vi "APS-7050 Wrapper.vi"(7 "States":T3=enum."Config", 8 "error in":errorcluster, 9 "Enable Output":bool=TRUE, 10 "Setting":T2, 11 "Alias":string="ACPS") -> (0 "error out":errorcluster, 1 "Connect?":bool, 2 "output cluster":T1, 3 "Measurement":dbl=nan)   [LabVIEW 2021, in "MIO Wrappers.lvlib"]
doc: "This is a wrapper to support Keysight N6700C."
uses:
  MIO Wrappers.lvlib
  Controls/PS States.ctl
  Load INI/Controls/Instruments_Data.ctl
  <instrlib>/APS-7000 Series/APS-7000 Series.lvlib
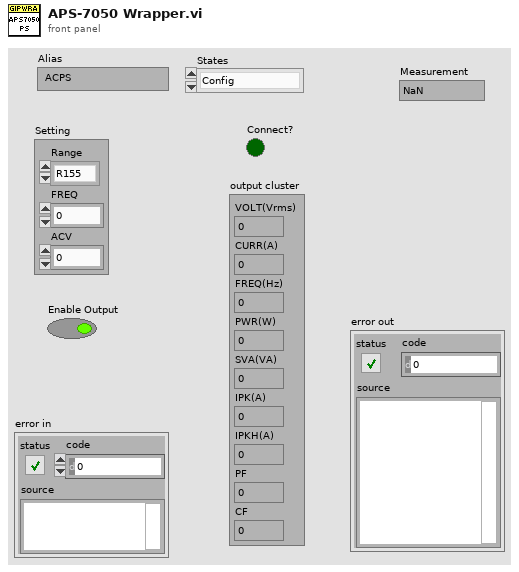
[diagram p1: front panel]
types:
  T1 = cluster{"VOLT(Vrms)":dbl, "CURR(A)":dbl, "FREQ(Hz)":dbl, "PWR(W)":dbl, "SVA(VA)":dbl, "IPK(A)":dbl, "IPKH(A)":dbl, "PF":dbl, "CF":dbl}
  T2 = cluster{"Range":enum16{"R155", "R310", "R600", "AUTO"}, "FREQ":dbl, "ACV":dbl}
  T3 = typedef "MIO Wrappers.lvlib/PS States.ctl" = enum16{"Init", "Config", "Enable Output", "Measure", "Close"}
  T4 = typedef "Instruments_Data.ctl" = cluster{"Alias":string, "Resource ":string}
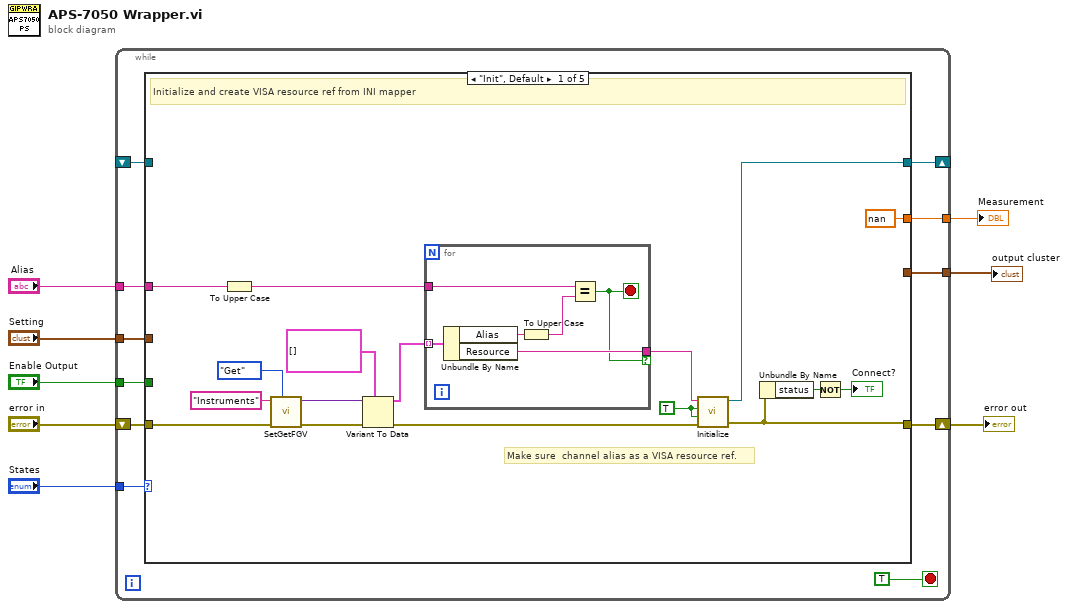
[diagram p0: block diagram]
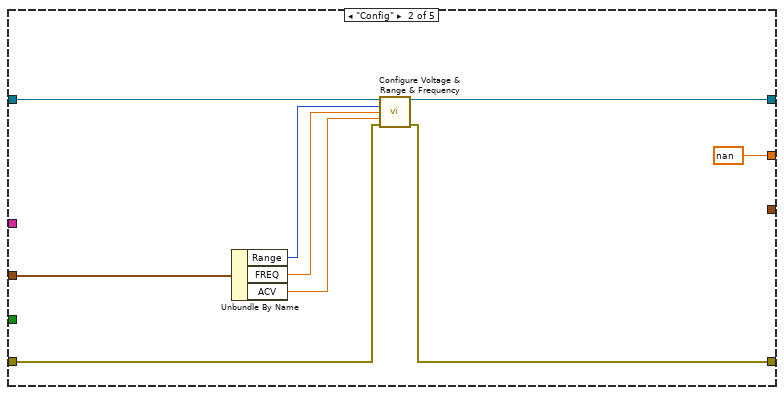
[diagram p2: hidden frame]
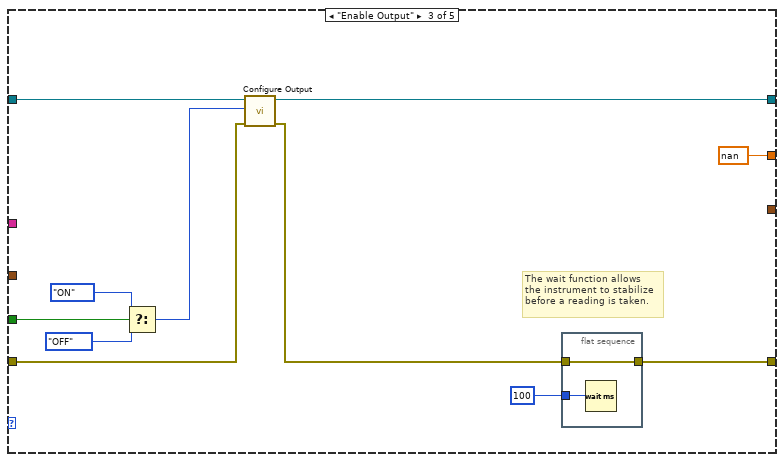
[diagram p3: hidden frame]
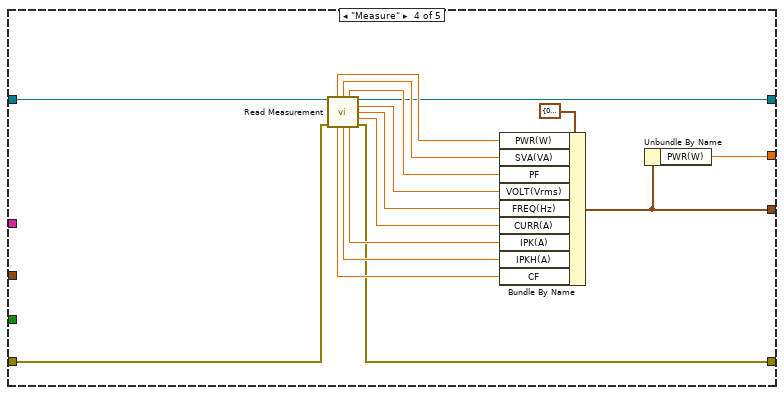
[diagram p4: hidden frame]
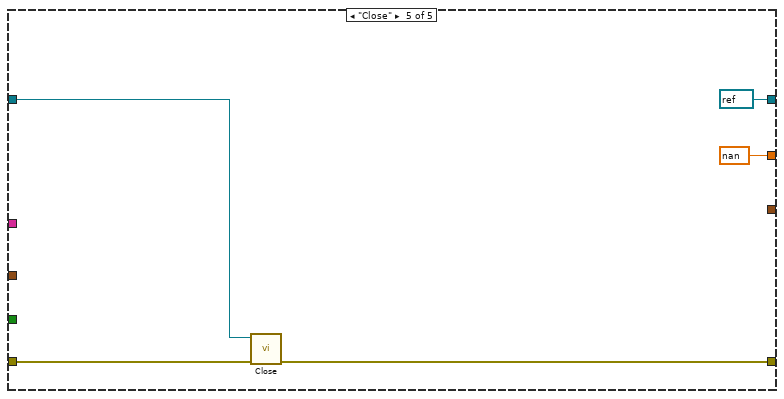
[diagram p5: hidden frame]
diagram:
  n1 = while {
    tunnel: "States" -> [w18]
    tunnel: "Enable Output" -> [w14]
    tunnel: "Setting" -> [w13]
    tunnel: [w11] -> w2
    shift-right: [w17] -> w6
    shift-left: "error in" -> [w19]
    shift-right: [w16] -> _
    shift-left: _ -> [w15]
    tunnel: "Alias" -> [w12]
    tunnel: [w9] -> w1
    stop <- TRUE stop-if-true
    n2 = case shown="\"Init\", Default" w18 {
      tunnel: w19 -> [w36 w50 w59 w70 w84]
      tunnel: [w22 w49 w62 w67 w83] -> w17
      tunnel: [w23 w47 w56 w68 refnum<visa-resource-name> refnum ("VISA out")] -> w16
      tunnel: w15 -> [_ w48 w57 w69 w82]
      tunnel: [nan nan nan w65 nan] -> w11
      tunnel: w14 -> [_ _ w55 _ _]
      tunnel: w13 -> [_ w46 _ _ _]
      tunnel: w12 -> [w30 _ _ _ _]
      tunnel: [_ _ _ w66 _] -> w9
      frame "Init", Default {
        w26 = TRUE ("ID Query (True)")
        # "Make sure  channel alias as a VISA resource ref."
        # "Initialize and create VISA resource ref from INI mapper"
        n3 = To Upper Case(1:w30) -> (0:w29:string)
        n4 = call "SetGetFGV.vi"("Method (Get)"=enum16{"Get", "Set"}."Get", "error in"=w36, "FGVname"="Instruments" ("Name")) -> ("error out"=w34:errorcluster, "Data out"=w33:variant)  [unwired: 7 in]
        n5 = Variant To Data(error in=w34, type=T4[] [], Variant=w33) -> (data=w31:T4[], error out=w25:errorcluster)
        n6 = for {
          tunnel: w31 -> [w42] mode=indexing
          tunnel: w29 -> [w41]
          tunnel: [w38] -> w24 if=w37
          stop <- w37 stop-if-true
          n7 = Unbundle By Name(w42) -> ("Alias"=w39:string, "Resource"=w38:string)
          n8 = To Upper Case(1:w39) -> (0:w40:string)
          n9 = Equal?(x=w41, y=w40) -> (x = y?=w37:bool)
        }
        n10 = call <instrlib>:"Initialize.vi"("error in (no error)"=w25, "Reset (True)"=w26, "ID Query (True)"=w26, "VISA resource name"=w24) -> ("error out"=w22:errorcluster, "VISA resource name out"=w23:refnum<visa-resource-name>)  [unwired: 6 in]
        n11 = Unbundle By Name(w22) -> ("status"=w21:bool)
        n12 = Not(x=w21) -> (.not. x?=→"Connect?":bool)
      }
      frame "Config" {
        n13 = Unbundle By Name(w46) -> ("Range"=w45:enum16{"R155", "R310", "R600", "AUTO"}, "FREQ"=w44:dbl, "ACV"=w43:dbl)
        n14 = call <instrlib>:"Configure Voltage & Range & Frequency.vi"("VISA in"=w48, "Range"=w45, "FREQ"=w44, "ACV"=w43, "error in"=w50) -> ("VISA out"=w47:refnum<visa-resource-name>, "error out"=w49:errorcluster)  [unwired: 2 in, 7 out]
      }
      frame "Enable Output" {
        # "The wait function allows \nthe instrument to stabilize\nbefore a reading is taken."
        n15 = Select(t=enum16{"OFF", "ON"}."ON" ("Output ON/OFF"), s=w55, f=enum16{"OFF", "ON"}."OFF" ("Output ON/OFF")) -> (s? t:f=w52:enum16{"OFF", "ON"})
        n16 = call <instrlib>:"Configure Output.vi"("error in"=w59, "Output ON/OFF"=w52, "VISA in"=w57) -> ("error out"=w58:errorcluster, "VISA out"=w56:refnum<visa-resource-name>)  [unwired: 6 in, 1 out]
        n17 = flat-sequence {
          tunnel: [w64] -> w62
          tunnel: w58 -> [w64]
          tunnel: u32 100 ("milliseconds to wait") -> [w63]
          frame #0 {
            n18 = Wait (ms)(milliseconds to wait=w63) -> ()  [unwired: 1 out]
          }
        }
      }
      frame "Measure" {
        n19 = call <instrlib>:"Read Measurement.vi"("VISA in"=w69, "error in"=w70) -> ("Power? (W)"=w77:dbl, "SVA? (VA)"=w76:dbl, "PF?"=w75:dbl, "VISA out"=w68:refnum<visa-resource-name>, "Vmeas? (Vrms)"=w74:dbl, "Fmeas? (Hz)"=w73:dbl, "Imeas? (Arms)"=w72:dbl, "Ipeak,hold?  (A)"=w80:dbl, "Ipeak? (A)"=w79:dbl, "CF?"=w78:dbl, "error out"=w67:errorcluster)  [unwired: 3 in]
        n20 = Bundle By Name(cluster=T1 {"VOLT(Vrms)"=0.0, "CURR(A)"=0.0, "FREQ(Hz)"=0.0, "PWR(W)"=0.0, "SVA(VA)"=0.0, "IPK(A)"=0.0, "IPKH(A)"=0.0, "PF"=0.0, "CF"=0.0} ("output cluster"), "PWR(W)"=w77, "SVA(VA)"=w76, "PF"=w75, "VOLT(Vrms)"=w74, "FREQ(Hz)"=w73, "CURR(A)"=w72, "IPK(A)"=w78, "IPKH(A)"=w79, "CF"=w80) -> (w66:T1)
        n21 = Unbundle By Name(w66) -> ("PWR(W)"=w65:dbl)
      }
      frame "Close" {
        n22 = call <instrlib>:"Close.vi"("error in (no error)"=w84, "VISA resource name"=w82) -> ("error out"=w83:errorcluster)  [unwired: 9 in]
      }
    }
  }
  "error out" <- w6
  "Measurement" <- w2
  "output cluster" <- w1
